vi "3_DrawScale (SubVI).vi"(6 "Scale colour":u32(colorbox)=16777225, 9 "N microns":dbl=500.0 format="%#_13g", 10 "um/pix":dbl, 11 "Refnum in":T1) -> (3 "Refnum out":T1)   [LabVIEW 2017]
uses:
  <vilib>/vision/Image Controls.llb/IMAQ Image.ctl
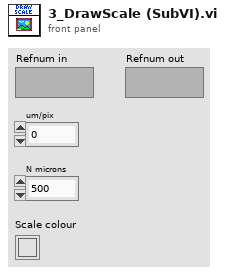
[diagram p1: front panel]
types:
  T1 = typedef "IMAQ Image.ctl" = refnum<image>
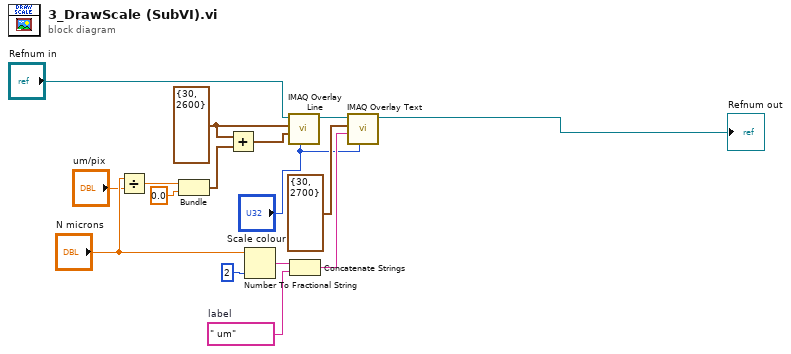
[diagram p0: block diagram]
diagram:
  w16 = " um"  # label
  w2 = cluster{"X":i32, "Y":i32} {"X"=30, "Y"=2600} ("Start Point")
  n1 = Divide(x="N microns", y="um/pix") -> (x/y=w6:dbl)
  n2 = Bundle(w6, "x"=0.0) -> (w4:cluster{dbl, "x":dbl})  [unwired: 1 in]
  n3 = Add(x=w2, y=w4) -> (x+y=w5:cluster{dbl, dbl})
  n4 = Number To Fractional String(number="N microns", precision (6)=i16 2) -> (F-format string=w14:string)  [unwired: 2 in]
  n5 = call "IMAQ Overlay Line"("Color"="Scale colour", "End Point"=w5, "Start Point"=w2, "Image"="Refnum in") -> ("Image Out"=w8:T1)  [unwired: 6 in, 1 out]
  n6 = Concatenate Strings(w14, w16) -> (w15:string)
  n7 = call "IMAQ Overlay Text"("Text Color (black)"="Scale colour", "String"=w15, "Origin"=cluster{"X":i32, "Y":i32} {"X"=30, "Y"=2700} ("Start Point"), "Image"=w8) -> ("Image Out"=→"Refnum out":T1)  [unwired: 6 in, 1 out]
